vi "P3-4.vi"() -> ()   [LabVIEW 2011]
panel:
  out "미터":dbl(knob) scale=0.0..10000.0
  out "불리언":bool
  in  "숫자형":dbl
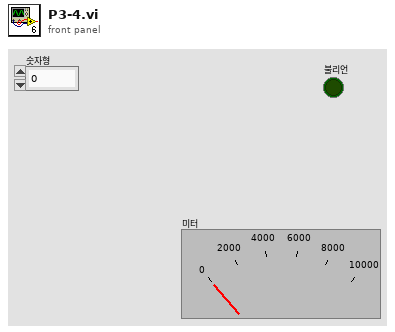
[diagram p1: front panel]
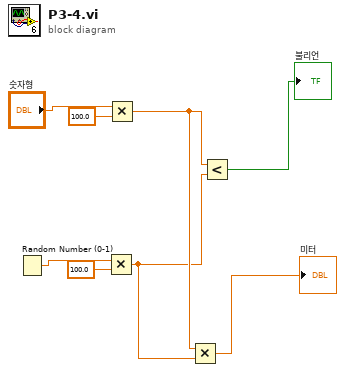
[diagram p0: block diagram]
diagram:
  n1 = Random Number (0-1)() -> (number: 0 to 1=w7:dbl)
  n2 = Multiply(x=w7, y=100.0) -> (x*y=w2:dbl)
  n3 = Multiply(x="숫자형", y=100.0) -> (x*y=w3:dbl)
  n4 = Multiply(x=w3, y=w2) -> (x*y=→"미터":dbl)
  n5 = Less?(x=w3, y=w2) -> (x < y?=→"불리언":bool)
